vi "DB_SelectData.vi"(8 "error in (no error)":errorcluster, 11 "SQLite Connection in":refnum<class "Connection.lvclass">) -> (0 "error out":errorcluster, 2 "Data":string[][](table), 3 "SQLite Connection":refnum<class "Connection.lvclass">)   [LabVIEW 2020]
doc: "Selects all of the data from the database."
uses:
  <vilib>/drjdpowell/SQLite Library/SQL Connection/Connection.lvclass
  <vilib>/drjdpowell/SQLite Library/SQL Statement/SQL Statement.lvclass/SQL Statement.ctl
  <vilib>/drjdpowell/SQLite Library/SQL Statement/Error Message.vi
  <vilib>/drjdpowell/SQLite Library/SQL Statement/Column String.vi
  <vilib>/drjdpowell/SQLite Library/SQL Statement/Column Timestamp.vi
  <vilib>/drjdpowell/SQLite Library/SQL Statement/SQL Statement.lvclass
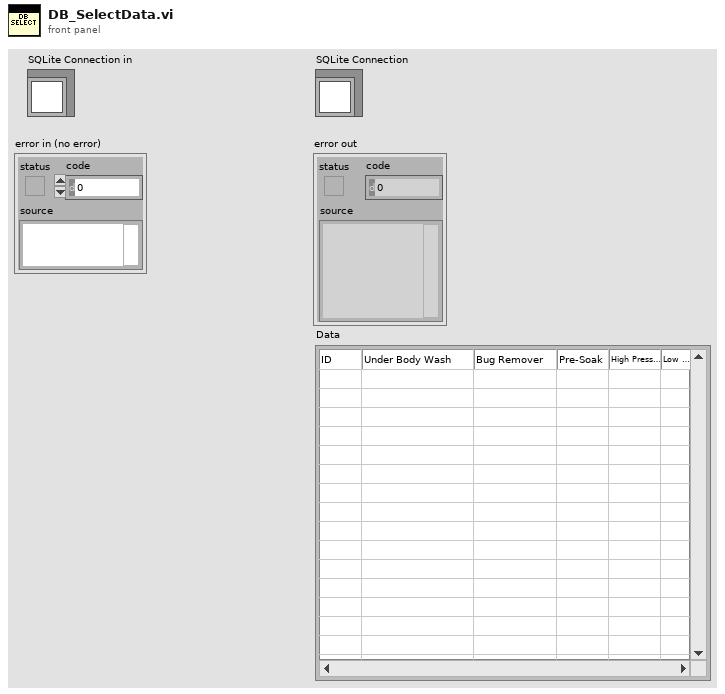
[diagram p1: front panel]
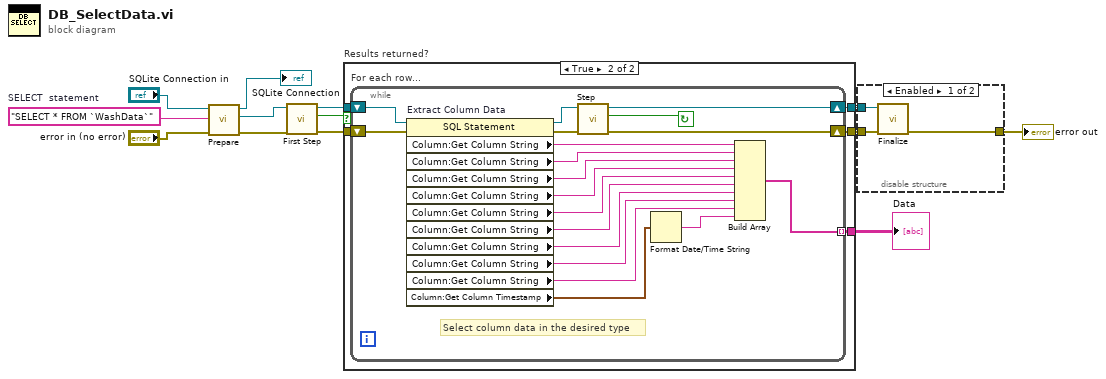
[diagram p0: block diagram]
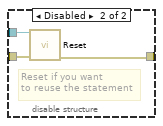
[diagram p2: hidden frame]
diagram:
  w11 = "SELECT * FROM `WashData`"  # SELECT  statement
  n1 = call <vilib>:"Prepare.vi"("error in (no error)"="error in (no error)", "SQL"=w11, "SQLite Connection in"="SQLite Connection in") -> ("error out"=w7:errorcluster, "SQL Statement"=w6:refnum<class "SQL Statement.lvclass">, "SQLite Connection"=→"SQLite Connection":refnum<class "Connection.lvclass">)  [unwired: 4 in, 2 out]
  n2 = call <vilib>:"First Step.vi"("error in (no error)"=w7, "SQL Statement in"=w6) -> ("error out"=w9:errorcluster, "Row returned"=w8:bool, "SQL Statement"=w10:refnum<class "SQL Statement.lvclass">)  [unwired: 7 in]
  n3 = case "Results returned?" shown="True" w8 {
    tunnel: [w15 w20] -> w12
    tunnel: [w14 w19] -> w13
    tunnel: w10 -> [w15 w18]
    tunnel: w9 -> [w14 w17]
    tunnel: [_ w16] -> w1
    frame False {
    }
    frame True {
      n4 = while "For each row..." {
        shift-right: [w38] -> w20
        shift-left: w18 -> [w35]
        shift-right: [w36] -> w19
        shift-left: w17 -> [w34]
        tunnel: [w30] -> w16 mode=indexing
        stop <- w33 continue-if-true
        # "Select column data in the desired type"
        n5 = property on="Extract Column Data" class="SQL Statement"(reference=w35, error in=w34) -> (reference out=w39:refnum<class "SQL Statement.lvclass">, error out=w37:errorcluster, "Column:Get Column String"=w32:string, "Column:Get Column String"=w31:string, "Column:Get Column String"=w28:string, "Column:Get Column String"=w27:string, "Column:Get Column String"=w26:string, "Column:Get Column String"=w25:string, "Column:Get Column String"=w24:string, "Column:Get Column String"=w23:string, "Column:Get Column String"=w22:string, "Column:Get Column Timestamp"=w29:timestamp)
        n6 = call <vilib>:"Step.vi"("error in (no error)"=w37, "SQL Statement in"=w39) -> ("error out"=w36:errorcluster, "Row returned"=w33:bool, "SQL Statement"=w38:refnum<class "SQL Statement.lvclass">)  [unwired: 7 in]
        n7 = Format Date/Time String(seconds (now)=w29) -> (date/time string=w21:string)  [unwired: 2 in]
        n8 = Build Array(w32, w31, w28, w27, w26, w25, w24, w23, w22, w21) -> (w30:string[])
      }
    }
  }
  "Data" <- w1
  n9 = disable-structure "Diagram Disable Structure" shown="Enabled" {
    disable-tunnel: w12 -> [w42 w45]
    disable-tunnel: w13 -> [w41 w44]
    disable-tunnel: [w40 w43] -> w3
    frame Enabled {
      n10 = call <vilib>:"Finalize.vi"("error in (no error)"=w41, "SQL Statement in"=w42) -> ("error out"=w40:errorcluster)  [unwired: 9 in]
    }
    frame Disabled {
      # "Reset if you want\nto reuse the statement"
      n11 = call <vilib>:"Reset.vi"("error in (no error)"=w44, "SQL Statement in"=w45) -> ("error out"=w43:errorcluster)  [unwired: 8 in, 1 out]
    }
  }
  "error out" <- w3
